vi "Hood Control.vi"(7 "Vision":bool, 8 "Top":T1, 9 "AIDeviceRef":T4, 11 "Bottom":T1) -> (0 "HoodSpeed":dbl, 1 "Voltage":dbl, 2 "Shoter Angle":dbl)   [LabVIEW 2011]
uses:
  <vilib>/Rock Robotics/WPI/DigitalInput/WPI_DigitalInputDevRef.ctl
  <vilib>/Rock Robotics/SystemInterfaces/DIO/FPGA_DIOChannel.ctl
  <vilib>/Rock Robotics/SystemInterfaces/Typedef/FPGA_TypedefDigitalModule.ctl
  <vilib>/Rock Robotics/WPI/AnalogChannel/WPI_AnalogChannelDevRef.ctl
  <vilib>/Rock Robotics/SystemInterfaces/Typedef/FPGA_TypedefAnalogModule.ctl
  <vilib>/Rock Robotics/SystemInterfaces/AI/FPGA_AIChannel.ctl
  System Set Points and States.vi
  Robot Global Data.vi
panel:
  out "Target Info[0].Distance (ft)":dbl
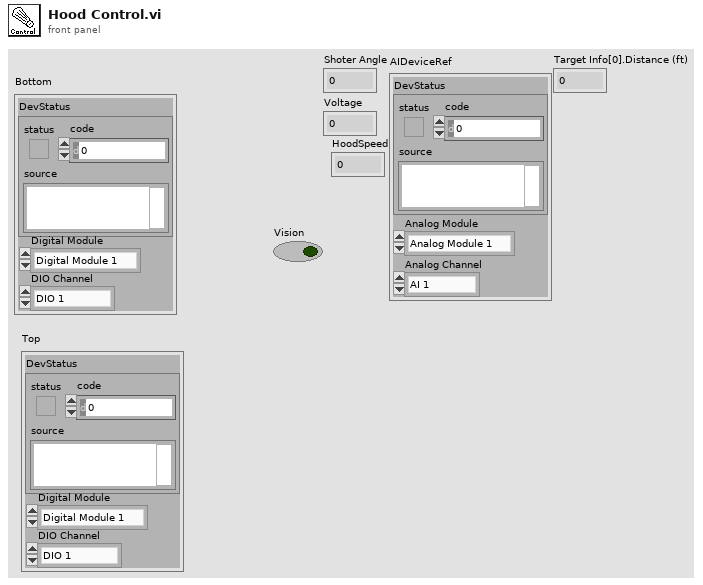
[diagram p1: front panel]
types:
  T1 = typedef "WPI_DigitalInputDevRef.ctl" = cluster{"DevStatus":errorcluster, "DIO Channel":T2, "Digital Module":T3}
  T2 = typedef "FPGA_DIOChannel.ctl" = enum8{"DIO 1", "DIO 2", "DIO 3", "DIO 4", "DIO 5", "DIO 6", "DIO 7", "DIO 8", "DIO 9", "DIO 10", "DIO 11", "DIO 12", "DIO 13", "DIO 14", "Invalid"}
  T3 = typedef "FPGA_TypedefDigitalModule.ctl" = enum16{"Digital Module 1", "Digital Module 2"}
  T4 = typedef "WPI_AnalogChannelDevRef.ctl" = cluster{"DevStatus":errorcluster, "Analog Module":T5, "Analog Channel":T6}
  T5 = typedef "FPGA_TypedefAnalogModule.ctl" = enum16{"Analog Module 1", "Analog Module 2"}
  T6 = typedef "FPGA_AIChannel.ctl" = enum8{"AI 1", "AI 2", "AI 3", "AI 4", "AI 5", "AI 6", "AI 7", "AI 8", "Invalid"}
  T7 = cluster{"Position":cluster{"X":dbl, "Y":dbl}, "Distance (ft)":dbl}[]
  T8 = cluster{"Target Info[0]":cluster{"Position":cluster{"X":dbl, "Y":dbl}, "Distance (ft)":dbl}, "Target Info[1]":cluster{"Position":cluster{"X":dbl, "Y":dbl}, "Distance (ft)":dbl}, "Target Info[2]":cluster{"Position":cluster{"X":dbl, "Y":dbl}, "Distance (ft)":dbl}, "Target Info[3]":cluster{"Position":cluster{"X":dbl, "Y":dbl}, "Distance (ft)":dbl}, "Target Info[4]":cluster{"Position":cluster{"X":dbl, "Y":dbl}, "Distance (ft)":dbl}, "Target Info[5]":cluster{"Position":cluster{"X":dbl, "Y":dbl}, "Distance (ft)":dbl}, "Target Info[6]":cluster{"Position":cluster{"X":dbl, "Y":dbl}, "Distance (ft)":dbl}, "Target Info[7]":cluster{"Position":cluster{"X":dbl, "Y":dbl}, "Distance (ft)":dbl}, "Target Info[8]":cluster{"Position":cluster{"X":dbl, "Y":dbl}, "Distance (ft)":dbl}}
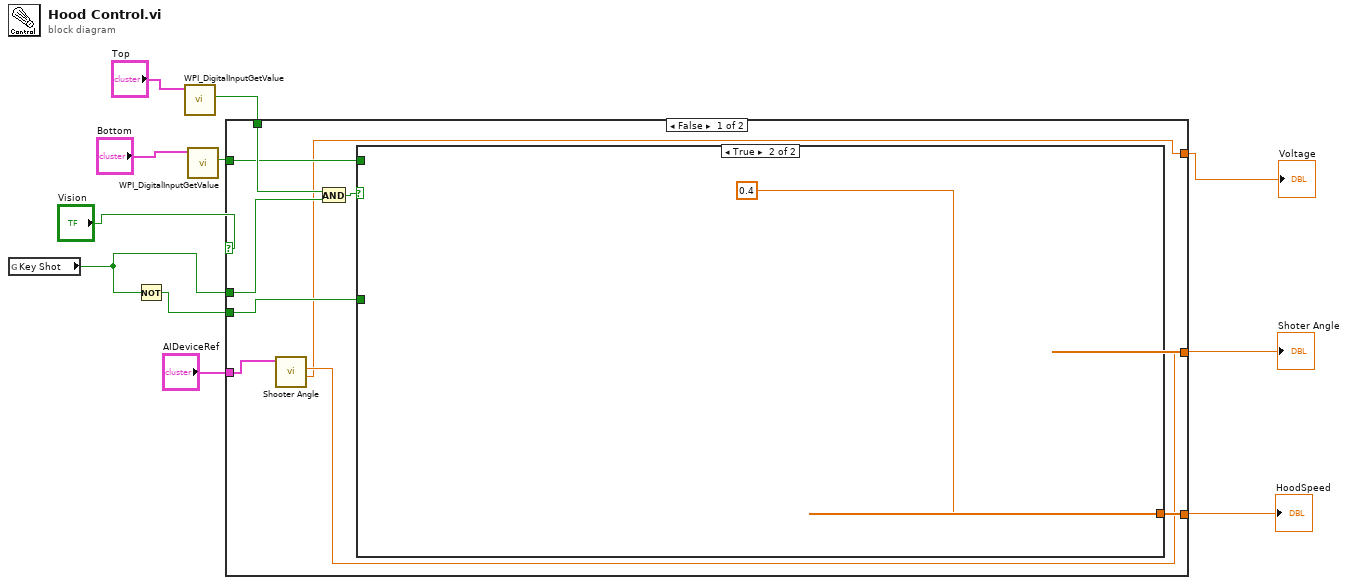
[diagram p0: block diagram]
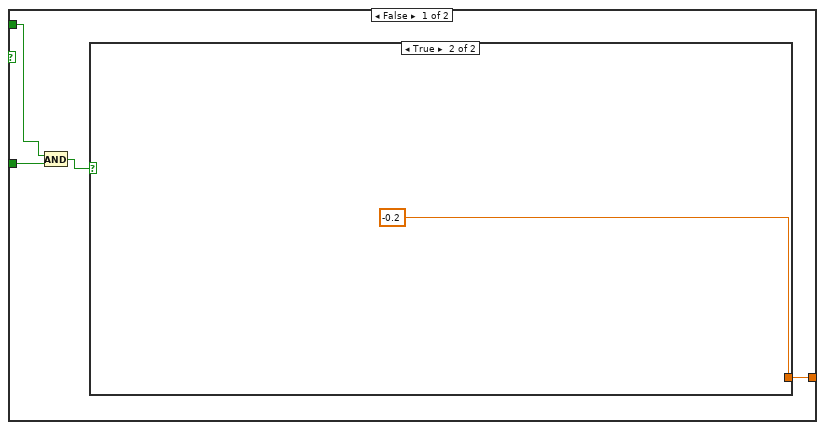
[diagram p2: hidden frame]
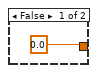
[diagram p3: hidden frame]
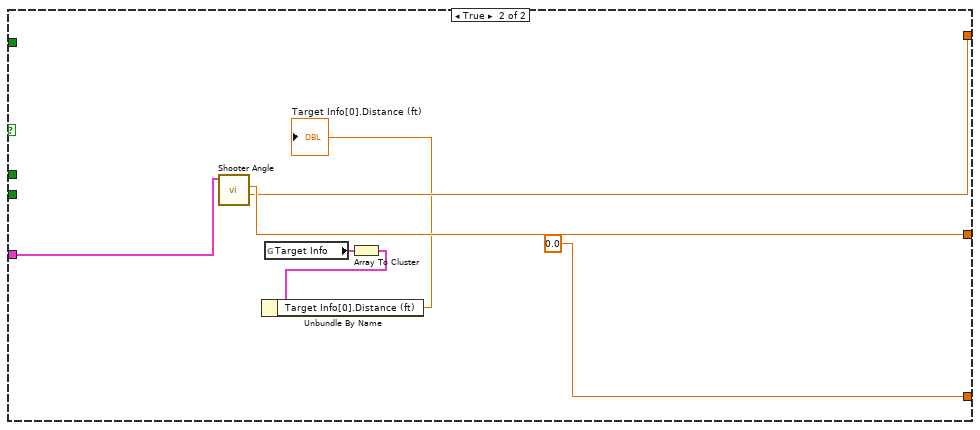
[diagram p4: hidden frame]
diagram:
  n1 = global read "System Set Points and States.vi" "Key Shot"() -> (w2:bool)
  n2 = Not(x=w2) -> (.not. x?=w1:bool)
  n3 = call <vilib>:"WPI_DigitalInputGetValue.vi"("DigitalInputDevRef"="Top") -> ("Value"=w3:bool)  [unwired: 8 in, 2 out]
  n4 = call <vilib>:"WPI_DigitalInputGetValue.vi"("DigitalInputDevRef"="Bottom") -> ("Value"=w8:bool)  [unwired: 8 in, 2 out]
  n5 = case shown="False" "Vision" {
    tunnel: w1 -> [w16 _]
    tunnel: w2 -> [w20 _]
    tunnel: [w17 0.0 ("Output")] -> w10
    tunnel: w8 -> [w15 _]
    tunnel: [w13 w34] -> w7
    tunnel: [w12 w33] -> w6
    tunnel: "AIDeviceRef" -> [w14 w32]
    tunnel: w3 -> [w19 _]
    frame False {
      n6 = call "Shooter Angle.vi"("AIDeviceRef"=w14) -> ("Voltage"=w12:dbl, "Shoter Angle"=w13:dbl)  [unwired: 9 in]
      n7 = And(x=w19, y=w20) -> (x .and. y?=w18:bool)
      n8 = case shown="True" w18 {
        tunnel: [w22 0.4 ("Voltage")] -> w17
        tunnel: w16 -> [w24 _]
        tunnel: w15 -> [w21 _]
        frame False {
          n9 = And(x=w21, y=w24) -> (x .and. y?=w23:bool)
          n10 = case shown="True" w23 {
            tunnel: [0.0 ("Voltage") -0.2 ("Voltage")] -> w22
            frame False {
            }
            frame True {
            }
          }
        }
        frame True {
        }
      }
    }
    frame True {
      n11 = call "Shooter Angle.vi"("AIDeviceRef"=w32) -> ("Voltage"=w33:dbl, "Shoter Angle"=w34:dbl)  [unwired: 9 in]
      n12 = global read "Robot Global Data.vi" "Target Info"() -> (w31:T7)
      n13 = Array To Cluster(array=w31) -> (cluster=w30:T8)
      n14 = Unbundle By Name(w30) -> ("Target Info[0].Distance (ft)"=→"Target Info[0].Distance (ft)":dbl)
    }
  }
  "Shoter Angle" <- w7
  "Voltage" <- w6
  "HoodSpeed" <- w10
